vi "GetTimeSubVI.vi"() -> (3 "Milliseconds":dbl)   [LabVIEW 2019]
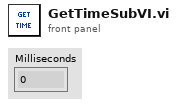
[diagram p1: front panel]
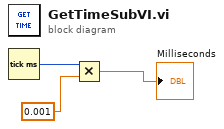
[diagram p0: block diagram]
diagram:
  n1 = Tick Count (ms)() -> (millisecond timer value=w1:u32)
  n2 = Multiply(x=w1, y=0.001) -> (x*y=→"Milliseconds":dbl)
